vi "Convert to Snake Case.vi"(8 "error in (no error)":errorcluster, 10 "All Upper Case? (F)":bool, 11 "Input String":string) -> (0 "error out":errorcluster, 3 "Output String":string)   [LabVIEW 2015, in "Case Manipulation.lvlib"]
doc: "Introduction:\nWe often remove the spaces between words because programs of different sorts reserve the space (‘ ’) character for special purposes. Because the space character is reserved, we cannot use it to represent a concept that we express in our human language with multiple words.\nSnake Case:\nThis style, when capitalized, is often used as a convention in declaring constants in many languages. When lower cased, it is used conventionally in declaring database field names."
uses:
  Case Manipulation.lvlib
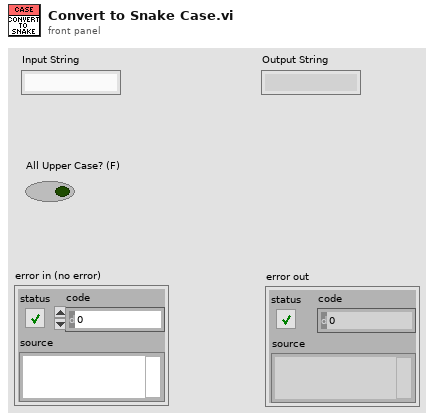
[diagram p1: front panel]
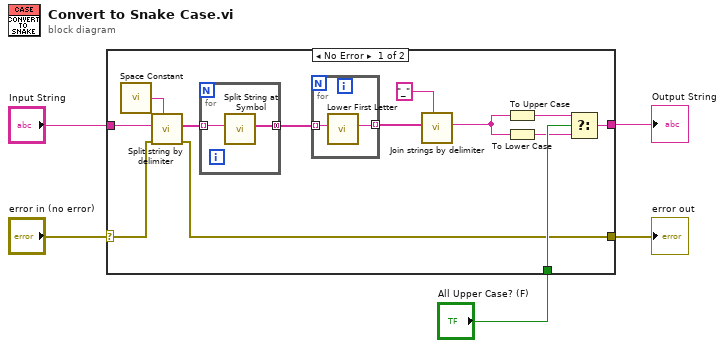
[diagram p0: block diagram]
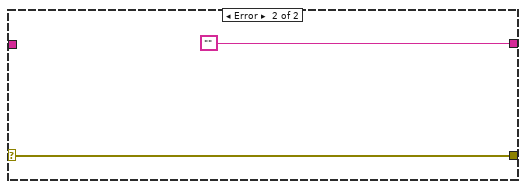
[diagram p2: hidden frame]
diagram:
  n1 = case shown="No Error" "error in (no error)" {
    selector: "error in (no error)" -> [w16 w24]
    tunnel: "Input String" -> [w18 _]
    tunnel: [w6 w24] -> w3
    tunnel: [w11 ""] -> w4
    tunnel: "All Upper Case? (F)" -> [w13 _]
    frame No Error {
      n2 = call <vilib>:"Space Constant.vi"() -> ("String"=w17:string)
      n3 = call "Split string by delimiter.vi"("Delimiter"=w17, "error in (no error)"=w16, "String In"=w18) -> ("error out"=w6:errorcluster, "String Array Out"=w8:string[])  [unwired: 7 in]
      n4 = for {
        tunnel: w8 -> [w20] mode=indexing
        tunnel: [w19] -> w7 mode=concatenating
        n5 = call "Split String at Symbol.vi"("String In"=w20) -> ("String Array Out"=w19:string[])  [unwired: 9 in, 1 out]
      }
      n6 = for {
        tunnel: w7 -> [w22] mode=indexing
        tunnel: [w21] -> w15 mode=indexing
        n7 = call "Lower First Letter.vi"("String In"=w22) -> ("String Out"=w21:string)  [unwired: 10 in]
      }
      n8 = call "Join strings by delimiter.vi"("Delimiter"="_", "Strings []"=w15) -> ("String Out"=w9:string)  [unwired: 9 in]
      n9 = To Upper Case(1:w9) -> (0:w12:string)
      n10 = To Lower Case(string=w9) -> (all lower case string=w10:string)
      n11 = Select(t=w12, s=w13, f=w10) -> (s? t:f=w11:string)
    }
    frame Error {
    }
  }
  "error out" <- w3
  "Output String" <- w4
